vi "subImagesAndBfiled.vi"(9 "B [T]":dbl, 11 "MagAnalysis_Online in":refnum<class "MagAnalysis_Online.lvclass">) -> (1 "B[T]":dbl, 2 "new ROI":bool, 3 "MagAnalysis_Online out":refnum<class "MagAnalysis_Online.lvclass">, 4 "Numeric 2":u32, 5 "OK":bool[](array[boolean]))   [LabVIEW 2011, in "MagAnalysis_Online.lvclass"]
uses:
  MagAnalysis_Online.lvclass
  bgImages_tyudef.ctl
  IMAQ Image.ctl
  MagAnalysis_Online.lvclass/MagAnalysis_Online.ctl
panel:
  out "BGImages":T1
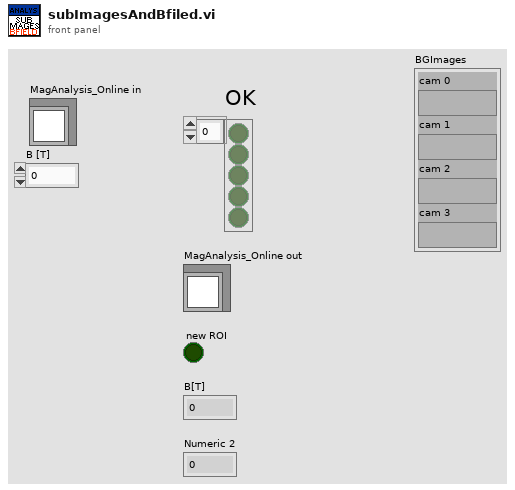
[diagram p1: front panel]
types:
  T1 = typedef "bgImages_tyudef.ctl" = cluster{"cam 0":T2, "cam 1":T2, "cam 2":T2, "cam 3":T2}
  T2 = typedef "IMAQ Image.ctl" = refnum<image>
  T3 = typedef "CamSettings_Typdef.ctl" = cluster{"Cam 0":T4, "Cam 1":T4, "Cam 2":T4, "Cam 3":T4}
  T4 = typedef "CamSettingSUB_TypDEf.ctl" = cluster{"position":dbl, "Field of view":dbl, "start":dbl, "end":dbl, "center":dbl, "Lens":T5, "Forward":T6, "Spec_Calib_file 2":path, "map":path, "y size":i32}
  T5 = typedef "CamAndObj_TypDEf.ctl" = enum16{"FL1-f8x08", "FL1-f8x06", "FL1-f8", "ch300-f50", "FL2G-f8", "FL3M14-f8", "FL3M14-f8x08", "FL3M14-f8x08(2x2)"}
  T6 = typedef "OnOffTypeDef.ctl" = enum16{"off", "on"}
  T7 = typedef "Calib_Typdef.ctl" = cluster{"cam 0":T8, "cam 1":T8, "cam 2":T8, "cam 3":T8}
  T8 = typedef "calib_Sub_Typdef.ctl" = cluster{"incident ANGLE COMPENSATION":dbl[], "field of view /pixel":dbl, "dp/B [MeV/C/B]":dbl[], "charge compensation":dbl[], "Momentum [MeV/C]":dbl[], "B [T]":dbl, "energyDependence Input":dbl[], "pixel angle (y)":dbl[], "dp [MeV/C/] ":dbl[], "angle 2Dfor spectrumj":dbl[][], "dp [MeV/C] 2D":dbl[][], "charge compensation 2D":dbl[][], "Screen&Camera 2":T9, "ROI info":T10, "Y 2D full angle":dbl[][]}
  T9 = typedef "ScreenCam2_TypDEf.ctl" = cluster{"Screen Orientation":string, "Screen angle":string, "Lens":T5, "Calibration (mm/pix)":dbl}
  T10 = typedef "ROIInfo_TypDef.ctl" = cluster{"npix-X":i32, "npix-Y":i32, "Left [pix]":dbl, "Top [pix]":dbl}
  T11 = typedef "SubscriberCluster_TypDEf.ctl" = cluster{"tcp data event":T12, "Event Registration Refnum":refnum<event-registration>, "data queue":refnum<queue>, "Devices":string[], "Alias":string[], "Variable header":string[], "Devices ALL":string[]}
  T12 = typedef "tcp_new_data_event.ctl" = refnum<user-event>
  T13 = typedef "MagAnalysis_Online.lvclass/analysis_data_typdef.ctl" = cluster{"cam0":T2, "cam1":T2, "cam2":T2, "cam3":T2}
  T14 = typedef "ROIStartfromCam_typdef.ctl" = cluster{"ROI 0":dbl, "ROI 1":dbl, "ROI 2":dbl, "ROI 3":dbl}
  T15 = typedef "dataTypdef.ctl" = cluster{"cam0":T2, "cam1":T2, "cam2":T2, "cam3":T2, "ROI 0":dbl, "ROI 1":dbl, "ROI 2":dbl, "ROI 3":dbl, "Bfield":dbl}
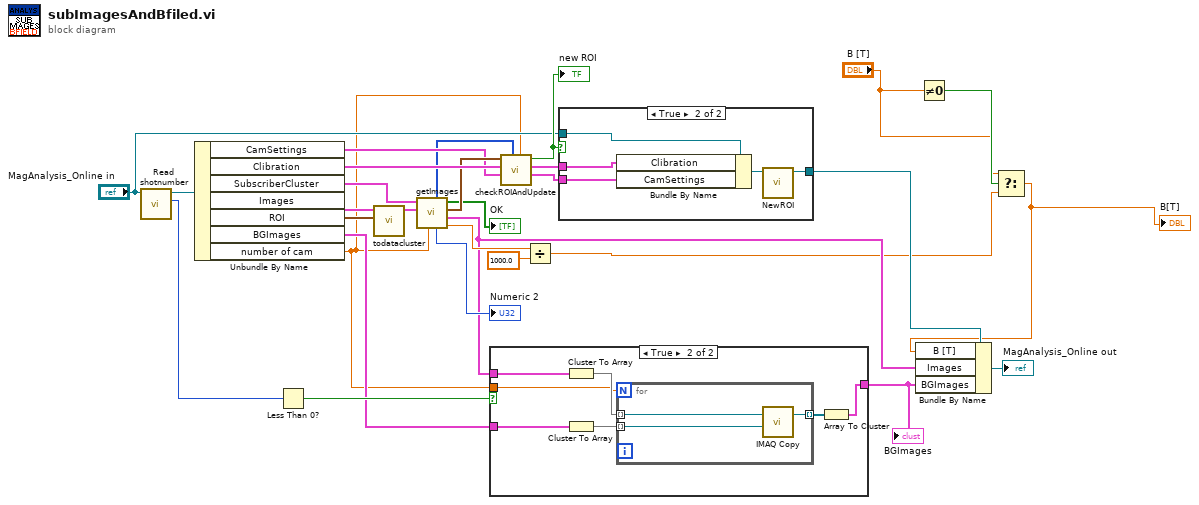
[diagram p0: block diagram]
diagram:
  n1 = call-dynamic "Read shotnumber.vi"("BaseDriver in"="MagAnalysis_Online in") -> ("shotnumber"=w15:i32, "BaseDriver out"=w14:refnum<class "MagAnalysis_Online.lvclass">)  [unwired: 7 in, 2 out]
  n2 = Unbundle By Name(w14) -> ("CamSettings"=w9:T3, "Clibration"=w29:T7, "SubscriberCluster"=w28:T11, "Images"=w25:T13, "ROI"=w26:T14, "BGImages"=w10:T1, "number of cam"=w5:dbl)
  n3 = Less Than 0?(x=w15) -> (x < 0?=w13:bool)
  n4 = call "todatacluster.vi"("ROI"=w26, "Images"=w25) -> ("data"=w27:T15)  [unwired: 9 in]
  n5 = call "getImages.vi"("Settings.number of cam"=w5, "data"=w27, "SubscriberCluster"=w28) -> ("B[mT]"=w22:dbl, "Images"=w12:T13, "ROI"=w18:T14, "OK"=→"OK":bool[], "Numeric"=→"Numeric 2":u32, "Y size"=w7:i32[])  [unwired: 3 in]
  n6 = case shown="True" w13 {
    tunnel: w12 -> [_ w37]
    tunnel: [w30 w32] -> w11
    tunnel: w10 -> [w30 w36]
    tunnel: w5 -> [_ w31]
    frame False {
    }
    frame True {
      n7 = Cluster To Array(cluster=w37) -> (array=w34:T2[])
      n8 = Cluster To Array(cluster=w36) -> (array=w35:T2[])
      n9 = for {
        N: w31 -> [_]
        tunnel: w35 -> [w40] mode=indexing
        tunnel: w34 -> [w39] mode=indexing
        tunnel: [w38] -> w33 mode=indexing
        n10 = call "IMAQ Copy"("Image Dst"=w40, "Image Src"=w39) -> ("Image Dst Out"=w38:T2)  [unwired: 4 in, 1 out]
      }
      n11 = Array To Cluster(array=w33) -> (cluster=w32:cluster{"[0]":T2, "[1]":T2, "[2]":T2, "[3]":T2})
    }
  }
  "BGImages" <- w11
  n12 = call "checkROIAndUpdate.vi"("Settings.number of cam"=w5, "Y size"=w7, "Settings.CamSettings 3"=w9, "Clibration"=w29, "ROI in"=w18) -> ("Settings.CamSettings 2"=w8:T3, "Clibration out"=w20:cluster{"[0]":T8, "[1]":T8, "[2]":T8, "[3]":T8}, "new ROI"=w19:bool)  [unwired: 4 in]
  "new ROI" <- w19
  n13 = Divide(x=w22, y=1000.0) -> (x/y=w2:dbl)
  n14 = case shown="True" w19 {
    tunnel: w20 -> [_ w46]
    tunnel: "MagAnalysis_Online in" -> [w41 w45]
    tunnel: [w41 w43] -> w23
    tunnel: w8 -> [_ w42]
    frame False {
    }
    frame True {
      n15 = Bundle By Name(cluster=w45, "Clibration"=w46, "CamSettings"=w42) -> (w44:refnum<class "MagAnalysis_Online.lvclass">)
      n16 = call "NewROI.vi"("MagAnalysis_Online in"=w44) -> ("MagAnalysis_Online out"=w43:refnum<class "MagAnalysis_Online.lvclass">)  [unwired: 10 in]
    }
  }
  n17 = Not Equal To 0?(x="B [T]") -> (x != 0?=w4:bool)
  n18 = Select(t="B [T]", s=w4, f=w2) -> (s? t:f=w1:dbl)
  "B[T]" <- w1
  n19 = Bundle By Name(cluster=w23, "B [T]"=w1, "Images"=w12, "BGImages"=w11) -> (→"MagAnalysis_Online out":refnum<class "MagAnalysis_Online.lvclass">)
